vi "getRampDataDAQ.vi"(8 "error in (no error)":errorcluster, 11 "ScriptEventList in":refnum<class "ScriptEventList.lvclass">) -> (0 "error out":errorcluster, 1 "data out":T1(array[cluster]), 2 "times out":dbl[](array[numeric]), 3 "ScriptEventList out":refnum<class "ScriptEventList.lvclass">)   [LabVIEW 2011, in "Tools.lvlib" / "Scripting.lvlib" / "ScriptEventList.lvclass"]
uses:
  ScriptEventList.lvclass
  DatabaseHelpers/Database Objects/Channel/Channel.lvclass
  ScriptEventList.lvclass/ScriptEventList.ctl
  ScriptEvent.lvclass
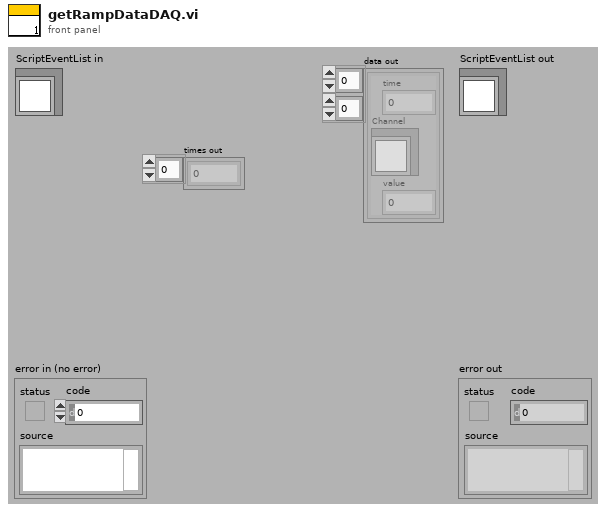
[diagram p1: front panel]
types:
  T1 = cluster{"time":dbl, "Channel":refnum<class "Channel.lvclass">, "value":dbl}[][]
  T2 = cluster{"times":dbl[], "Channel":refnum<class "Channel.lvclass">, "data":dbl[]}
  T3 = cluster{dbl, "Channel":refnum<class "Channel.lvclass">, dbl}[][]
  T4 = cluster{"time":dbl, "Channel":refnum<class "Channel.lvclass">, "data":dbl}[][]
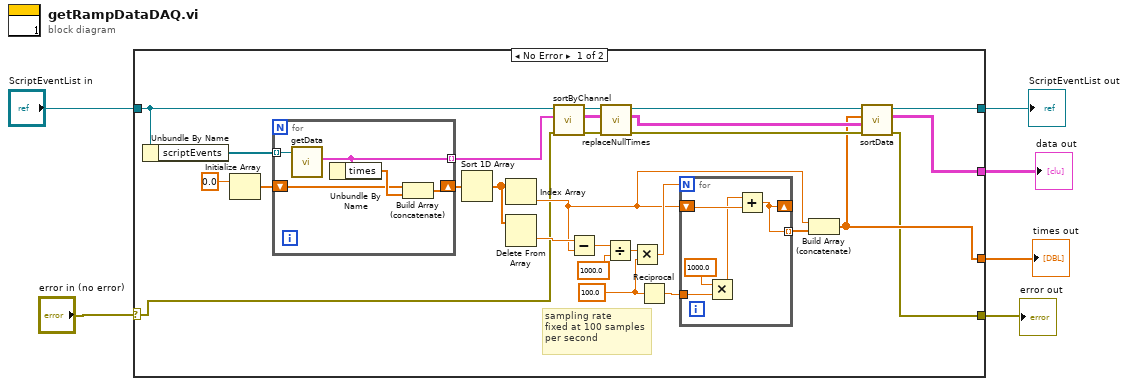
[diagram p0: block diagram]
diagram:
  n1 = case shown="No Error" "error in (no error)" {
    selector: "error in (no error)" -> [w8 w45]
    tunnel: [w7 w45] -> w5
    tunnel: [w23 w44] -> w3
    tunnel: "ScriptEventList in" -> [w9 w44]
    tunnel: [w10 _] -> w2
    tunnel: [w22 _] -> w1
    frame No Error {
      w15 = 100.0
      # "sampling rate\nfixed at 100 samples\nper second"
      n2 = Unbundle By Name(w9) -> ("scriptEvents"=w33:refnum<class "ScriptEvent.lvclass">[])
      n3 = Initialize Array(0.0) -> (w32:dbl[])  [unwired: 1 in]
      n4 = for {
        tunnel: w33 -> [w43] mode=indexing
        shift-right: [w41] -> w21
        shift-left: w32 -> [w40]
        tunnel: [w39] -> w30 mode=indexing
        n5 = call-dynamic "getData.vi"("ScriptEvent in"=w43) -> ("data"=w39:T2)  [unwired: 7 in, 3 out]
        n6 = Unbundle By Name(w39) -> ("times"=w42:dbl[])
        n7 = Build Array (concatenate)(w40, w42) -> (w41:dbl[])
      }
      n8 = Sort 1D Array(array=w21) -> (sorted array=w20:dbl[])
      n9 = Index Array(array=w20) -> (element=w11:dbl)  [unwired: 1 in]
      n10 = Delete From Array(array=w20) -> (deleted portion=w19:dbl)  [unwired: 2 in, 1 out]
      n11 = call "sortByChannel.vi"("error in (no error)"=w8, "Array"=w30, "ScriptEventList in"=w9) -> ("error out"=w27:errorcluster, "data"=w28:T3, "ScriptEventList out"=w29:refnum<class "ScriptEventList.lvclass">)  [unwired: 6 in]
      n12 = Subtract(x=w19, y=w11) -> (x-y=w18:dbl)
      n13 = call "replaceNullTimes.vi"("error in (no error)"=w27, "data in"=w28, "ScriptEventList in"=w29) -> ("error out"=w24:errorcluster, "data out"=w25:T1, "ScriptEventList out"=w26:refnum<class "ScriptEventList.lvclass">)  [unwired: 6 in]
      n14 = Divide(x=w18, y=1000.0) -> (x/y=w16:dbl)
      n15 = Multiply(x=w16, y=w15) -> (x*y=w13:dbl)
      n16 = Reciprocal(x=w15) -> (1/x=w14:dbl)
      n17 = for {
        N: w13 -> [_]
        tunnel: w14 -> [w37]
        tunnel: [w34] -> w12 mode=indexing
        shift-right: [w34] -> _
        shift-left: w11 -> [w38]
        n18 = Multiply(x=1000.0, y=w37) -> (x*y=w35:dbl)
        n19 = Add(x=w35, y=w38) -> (x+y=w34:dbl)
      }
      n20 = Build Array (concatenate)(w11, w12) -> (w10:dbl[])
      n21 = call "sortData.vi"("error in (no error)"=w24, "data"=w25, "times"=w10, "ScriptEventList in"=w26) -> ("error out"=w7:errorcluster, "data out"=w22:T4, "ScriptEventList out"=w23:refnum<class "ScriptEventList.lvclass">)  [unwired: 5 in]
    }
    frame Error {
    }
  }
  "error out" <- w5
  "ScriptEventList out" <- w3
  "times out" <- w2
  "data out" <- w1
